vi "Get Links.vi"(8 "error in (no error)":errorcluster, 11 "Robot Arm in":refnum<class "Robot Arm.lvclass">) -> (0 "error out":errorcluster, 2 "Links":refnum<class "Link.lvclass">[](array[class]), 3 "Robot Arm out":refnum<class "Robot Arm.lvclass">)   [LabVIEW 2013, in "Robot Arm.lvclass"]
uses:
  Robot Arm.lvclass
  Link/Link.lvclass
  Robot Arm.lvclass/Robot Arm.ctl
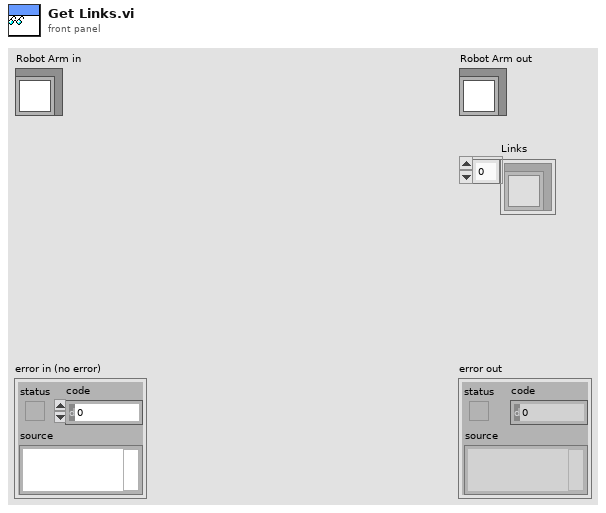
[diagram p1: front panel]
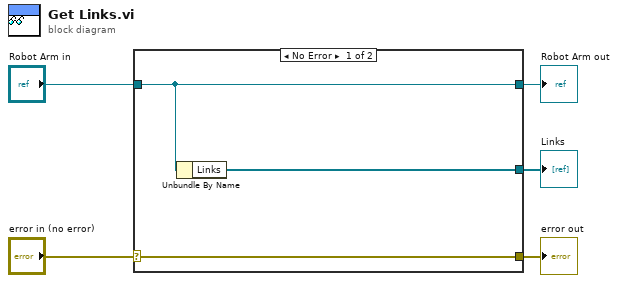
[diagram p0: block diagram]
diagram:
  n1 = case shown="No Error" "error in (no error)" {
    selector: "error in (no error)" -> [w8 w9]
    tunnel: [w8 w9] -> w4
    tunnel: [w7 w10] -> w2
    tunnel: "Robot Arm in" -> [w7 w10]
    tunnel: [w6 _] -> w1
    frame No Error {
      n2 = Unbundle By Name(w7) -> ("Links"=w6:refnum<class "Link.lvclass">[])
    }
    frame Error {
    }
  }
  "error out" <- w4
  "Robot Arm out" <- w2
  "Links" <- w1
